vi "Open.vi"(8 "error in (no error)":errorcluster, 11 "OBS in":refnum<class "OBS.lvclass">) -> (0 "error out":errorcluster, 3 "OBS out":refnum<class "OBS.lvclass">)   [LabVIEW 2020, in "obs-websocket.lvlib" / "OBS.lvclass"]
uses:
  OBS.lvclass
  Command.ctl
  OBS.lvclass/OBS.ctl
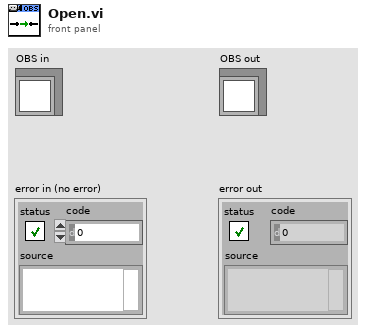
[diagram p1: front panel]
types:
  T1 = typedef "obs-websocket.lvlib/OBS.lvclass/Command.ctl" = enum16{"Open", "Close", "Stop"}
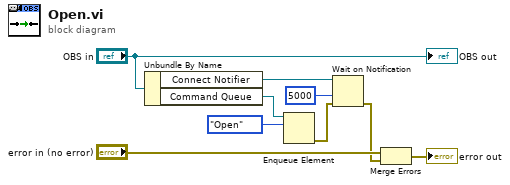
[diagram p0: block diagram]
diagram:
  n1 = Unbundle By Name("OBS in") -> ("Connect Notifier"=w7:refnum<notifier>, "Command Queue"=w9:refnum<queue>)
  n2 = Enqueue Element(queue=w9, element=Command."Open") -> (error out=w6:errorcluster)  [unwired: 2 in, 2 out]
  n3 = Wait on Notification(notifier=w7, timeout in ms (-1)=5000, error in (no error)=w6) -> (error out=w3:errorcluster)  [unwired: 1 in, 3 out]
  n4 = Merge Errors("error in (no error)", w3) -> (→"error out":errorcluster)
  "OBS out" <- "OBS in"
